vi "Shortest Distance Algorithm.vi"(2 "Speed":dbl, 3 "Motor Reversed?":bool, 4 "Encoder Angle":dbl(knob) scale=0.0..360.0, 5 "Setpoint":dbl(knob) scale=0.0..360.0) -> (0 "Reverse Motor":bool, 1 "PID Input":dbl(knob) scale=-180.0..180.0)   [LabVIEW 2016]
doc: "Inputs:\nSetpoint: Angle setpoint [0,360]\nEncoder Angle: Current wheel angle [0,360]\n\nOutput:\nPID Input: Difference between setpoint and wheel angle. Negative means turning clockwise is shorter, and positive means turning counterclockwise is shorter. [-180,180]"
uses:
  Swerve Global Variables.vi
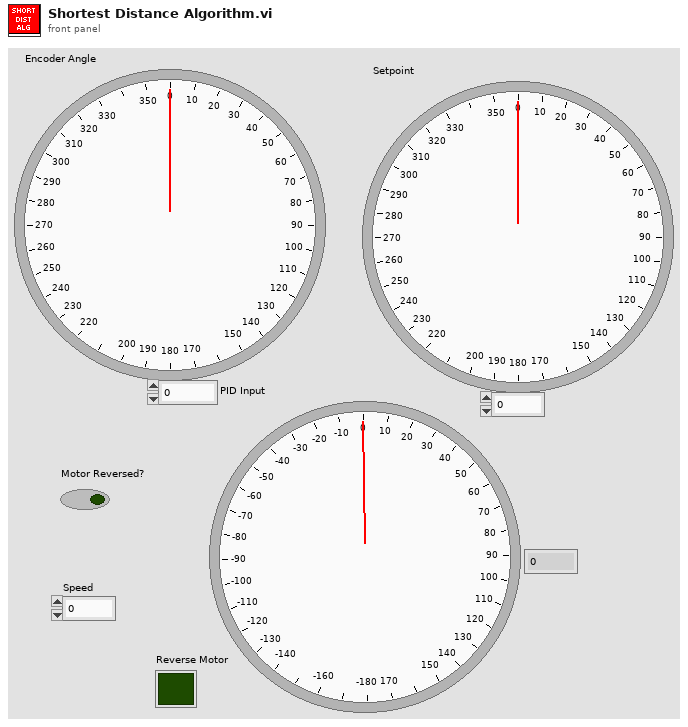
[diagram p1: front panel]
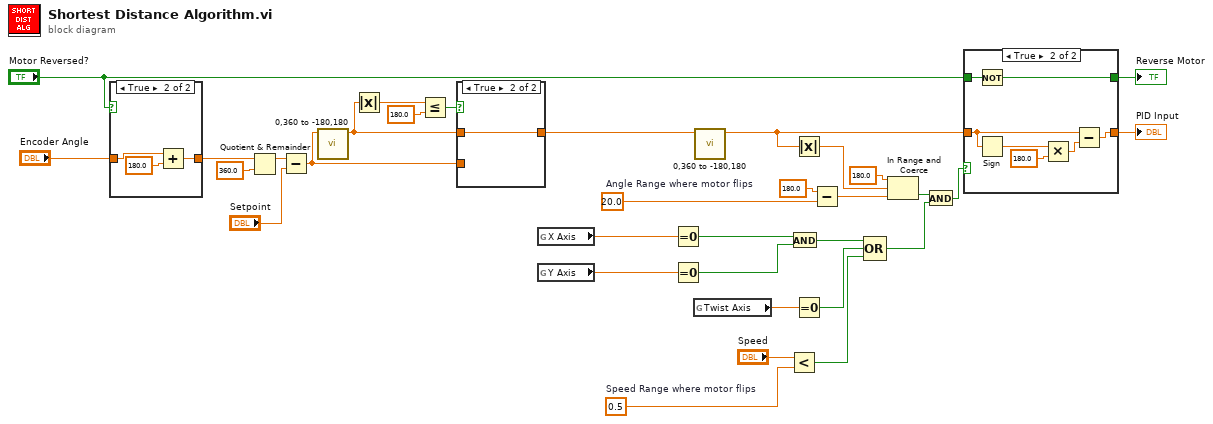
[diagram p0: block diagram]
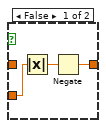
[diagram p4: hidden frame]
diagram:
  w2 = 0.5  # Speed Range where motor flips
  w24 = 20.0  # Angle Range where motor flips
  n1 = case shown="True" "Motor Reversed?" {
    tunnel: "Encoder Angle" -> [w34 w36]
    tunnel: [w34 w35] -> w18
    frame False {
    }
    frame True {
      n2 = Add(x=w36, y=180.0) -> (x+y=w35:dbl)
    }
  }
  n3 = Quotient & Remainder(x=w18, y=360.0) -> (x-y*floor(x/y)=w17:dbl)  [unwired: 1 out]
  n4 = Subtract(x=w17, y="Setpoint") -> (x-y=w28:dbl)
  n5 = call "0,360 to -180,180.vi"("Input [0,360]"=w28) -> ("Output [-180,180]"=w32:dbl)  [unwired: 10 in]
  n6 = Absolute Value(x=w32) -> (abs(x)=w30:dbl)
  n7 = Less Or Equal?(x=w30, y=180.0) -> (x <= y?=w33:bool)
  n8 = case shown="True" w33 {
    tunnel: [w38 w41] -> w27
    tunnel: w32 -> [_ w41]
    tunnel: w28 -> [w40 _]
    frame False {
      n9 = Absolute Value(x=w40) -> (abs(x)=w39:dbl)
      n10 = Negate(x=w39) -> (-x=w38:dbl)
    }
    frame True {
    }
  }
  n11 = global read "Swerve Global Variables.vi" "X Axis"() -> (w11:dbl)
  n12 = global read "Swerve Global Variables.vi" "Y Axis"() -> (w10:dbl)
  n13 = Equal To 0?(x=w11) -> (x = 0?=w8:bool)
  n14 = Equal To 0?(x=w10) -> (x = 0?=w7:bool)
  n15 = global read "Swerve Global Variables.vi" "Twist Axis"() -> (w9:dbl)
  n16 = call "0,360 to -180,180.vi"("Input [0,360]"=w27) -> ("Output [-180,180]"=w21:dbl)  [unwired: 10 in]
  n17 = Less?(x="Speed", y=w2) -> (x < y?=w1:bool)
  n18 = And(x=w8, y=w7) -> (x .and. y?=w6:bool)
  n19 = Absolute Value(x=w21) -> (abs(x)=w22:dbl)
  n20 = Equal To 0?(x=w9) -> (x = 0?=w5:bool)
  n21 = Subtract(x=180.0 ("upper limit"), y=w24) -> (x-y=w23:dbl)
  n22 = Compound Arithmetic op=OR(w6, w5, w1) -> (w4:bool)
  n23 = In Range and Coerce(upper limit=180.0, x=w22, lower limit=w23) -> (In Range?=w13:bool)  [unwired: 1 out]
  n24 = And(x=w13, y=w4) -> (x .and. y?=w12:bool)
  n25 = case shown="True" w12 {
    tunnel: w21 -> [w43 w47]
    tunnel: [w43 w46] -> w20
    tunnel: "Motor Reversed?" -> [w42 w45]
    tunnel: [w42 w44] -> w15
    frame False {
    }
    frame True {
      n26 = Not(x=w45) -> (.not. x?=w44:bool)
      n27 = Sign(1:w47) -> (0:w50:dbl)
      n28 = Multiply(x=w50, y=180.0) -> (x*y=w48:dbl)
      n29 = Subtract(x=w47, y=w48) -> (x-y=w46:dbl)
    }
  }
  "PID Input" <- w20
  "Reverse Motor" <- w15
